vi "Get Formatted Length.vi"(10 "delimiter":string, 11 "call chain":string[](array[string])) -> (3 "formatted length":u32)   [LabVIEW 2018, in "Logging.lvlib" / "Format String.lvclass"]
uses:
  Format String.lvclass
panel:
  # "Connector Pane"
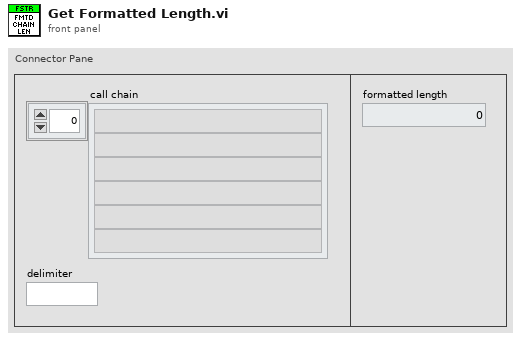
[diagram p1: front panel]
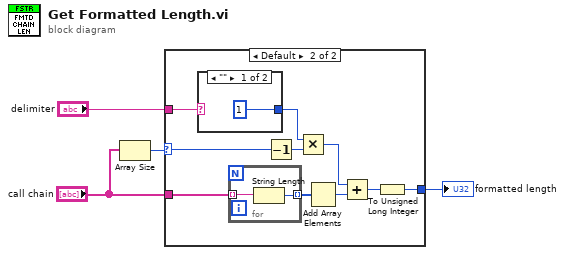
[diagram p0: block diagram]
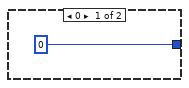
[diagram p2: hidden frame]
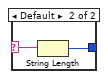
[diagram p3: hidden frame]
diagram:
  n1 = Array Size(array="call chain") -> (size(s)=w1:i32)
  n2 = case shown="Default" w1 {
    selector: w1 -> [_ w7]
    tunnel: [u32 0 w6] -> w4
    tunnel: "delimiter" -> [_ w10]
    tunnel: "call chain" -> [_ w9]
    frame 0 {
    }
    frame Default {
      n3 = case shown="\"\"" w10 {
        selector: w10 -> [_ w17]
        tunnel: [1 w18] -> w12
        frame "" {
        }
        frame Default {
          n4 = String Length(string=w17) -> (length=w18:i32)
        }
      }
      n5 = for {
        tunnel: w9 -> [w20] mode=indexing
        tunnel: [w19] -> w8 mode=indexing
        n6 = String Length(string=w20) -> (length=w19:i32)
      }
      n7 = Decrement(x=w7) -> (x-1=w11:i32)
      n8 = Multiply(x=w12, y=w11) -> (x*y=w14:i32)
      n9 = Add Array Elements(numeric array=w8) -> (sum=w13:i32)
      n10 = Add(x=w14, y=w13) -> (x+y=w15:i32)
      n11 = To Unsigned Long Integer(number=w15) -> (unsigned 32bit integer=w6:u32)
    }
  }
  "formatted length" <- w4
